vi "Variant to Attribute.vi"(8 "error in (no error)":errorcluster, 10 "Parameter":variant, 11 "CS++LNAReturnMessage in":refnum<class "CS++LNAReturnMessage.lvclass">) -> (0 "error out":errorcluster, 3 "CS++LNAReturnMessage out":refnum<class "CS++LNAReturnMessage.lvclass">)   [LabVIEW 2016, in "CS++LNA.lvlib" / "CS++LNAReturnMessage.lvclass"]
doc: "Read message attributes from parameter variant.\n\n<b>Attention:</b> This dynamic dispatch VI was added to the Message.lvclass in order to provide a mechnism to allow for generic parameter parsing. Refer to CS++LNA.lvlib:CS++LNAMessage.lvclass.Do.vi"
uses:
  CS++LNAReturnMessage.lvclass
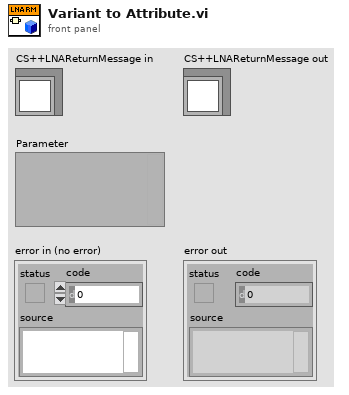
[diagram p1: front panel]
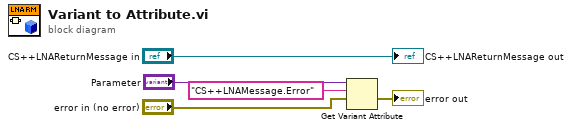
[diagram p0: block diagram]
diagram:
  n1 = Get Variant Attribute(Variant="Parameter", name="CS++LNAMessage.Error", default value (empty Variant)="error in (no error)") -> (value=→"error out":errorcluster)  [unwired: 1 in, 3 out]
  "CS++LNAReturnMessage out" <- "CS++LNAReturnMessage in"
